vi "moyennage.vi"(8 "Nb de valeurs par moyenne":i32, 11 "DSP Amplitude":dbl[](array[numeric])) -> (3 "DSP Amplitude Moyenné":dbl[](array[numeric]))   [LabVIEW 2017]
doc: "Sous-vi permettant de moyenner un vecteur X en sous plage."
uses:
  <vilib>/Analysis/baseanly.llb/Mean (DBL).vi
  variable_stop_globale.vi
  <vilib>/Analysis/NI_AALBase.lvlib
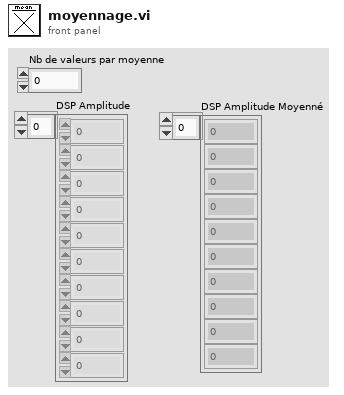
[diagram p1: front panel]
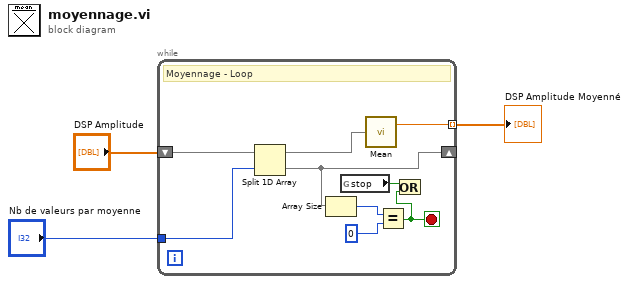
[diagram p0: block diagram]
diagram:
  n1 = while "Boucle While" {
    tunnel: [w10] -> w3 mode=indexing
    tunnel: "Nb de valeurs par moyenne" -> [w9]
    shift-right: [w7] -> _
    shift-left: "DSP Amplitude" -> [w8]
    stop <- w5 stop-if-true
    # "Moyennage - Loop"
    n2 = Split 1D Array(array=w8, index=w9) -> (first subarray=w6:dbl[], second subarray=w7:dbl[])
    n3 = Array Size(array=w7) -> (size(s)=w12:i32)
    n4 = global read "variable_stop_globale.vi" "stop"() -> (w4:bool)
    n5 = call-poly <vilib>:"Mean.vi"("X"=w6) -> ("mean"=w10:dbl)  [unwired: 1 out]
    n6 = Equal?(x=w12, y=0) -> (x = y?=w5:bool)
    n7 = Or(x=w4, y=w5) -> ()  [unwired: 1 out]
  }
  "DSP Amplitude Moyenné" <- w3
